vi "Live.vi"(1 "baud rate (9600)":u32=9600, 2 "VISA Resource (read)":refnum<visa-resource-name>="COM2") -> (0 "CAR DATA":T1)   [LabVIEW 2014]
uses:
  Program Files (x86)/National Instruments/LabVIEW 2014/examples/Instrument IO/Serial/support/Serial - Settings.ctl
  Type Def/CAR Data Cluster.ctl
  <vilib>/Instr/_visa.llb/VISA Configure Serial Port (Instr).vi
panel:
  in  "Termination Character":u8=10 format="%.0x"
  in  "End Write on Termination Character?":bool=TRUE
  in  "End Read on Termination Character?":bool=TRUE
  in  "Write String":string="*IDN?"
  in  "Serial Settings (read)":T2={"baud rate"=9600, "data bits"=8, "parity"=enum."None", "stop bits"=10, "flow control"=0} {"flow control" items=["None"=0, "XON/XOFF"=1, "RTS/CTS"=2, "DTR/DSR"=4]; "stop bits" items=["1.0"=10, "1.5"=15, "2.0"=20]; "data bits" min=5 max=8 step=1; "baud rate" items=["75"=75, "110"=110, "134"=134, "150"=150, "300"=300, "600"=600, "1200"=1200, "1800"=1800, "2400"=2400, "4800"=4800, "7200"=7200, "9600"=9600, "14400"=14400, "19200"=19200, "28800"=28800, "38400"=38400, "56000"=56000, "57600"=57600, "115200"=115200, "128000"=128000, "230400"=230400]}
  in  "Serial Settings (write)":T2={"baud rate"=9600, "data bits"=8, "parity"=enum."None", "stop bits"=10, "flow control"=0} {"flow control" items=["None"=0, "XON/XOFF"=1, "RTS/CTS"=2, "DTR/DSR"=4]; "stop bits" items=["1.0"=10, "1.5"=15, "2.0"=20]; "data bits" min=5 max=8 step=1; "baud rate" items=["75"=75, "110"=110, "134"=134, "150"=150, "300"=300, "600"=600, "1200"=1200, "1800"=1800, "2400"=2400, "4800"=4800, "7200"=7200, "9600"=9600, "14400"=14400, "19200"=19200, "28800"=28800, "38400"=38400, "56000"=56000, "57600"=57600, "115200"=115200, "128000"=128000, "230400"=230400]}
  in  "VISA Resource (write)":refnum<visa-resource-name>="COM1"
  out "bytes written":u32
  out "Read String":string
  out "bytes read":u32
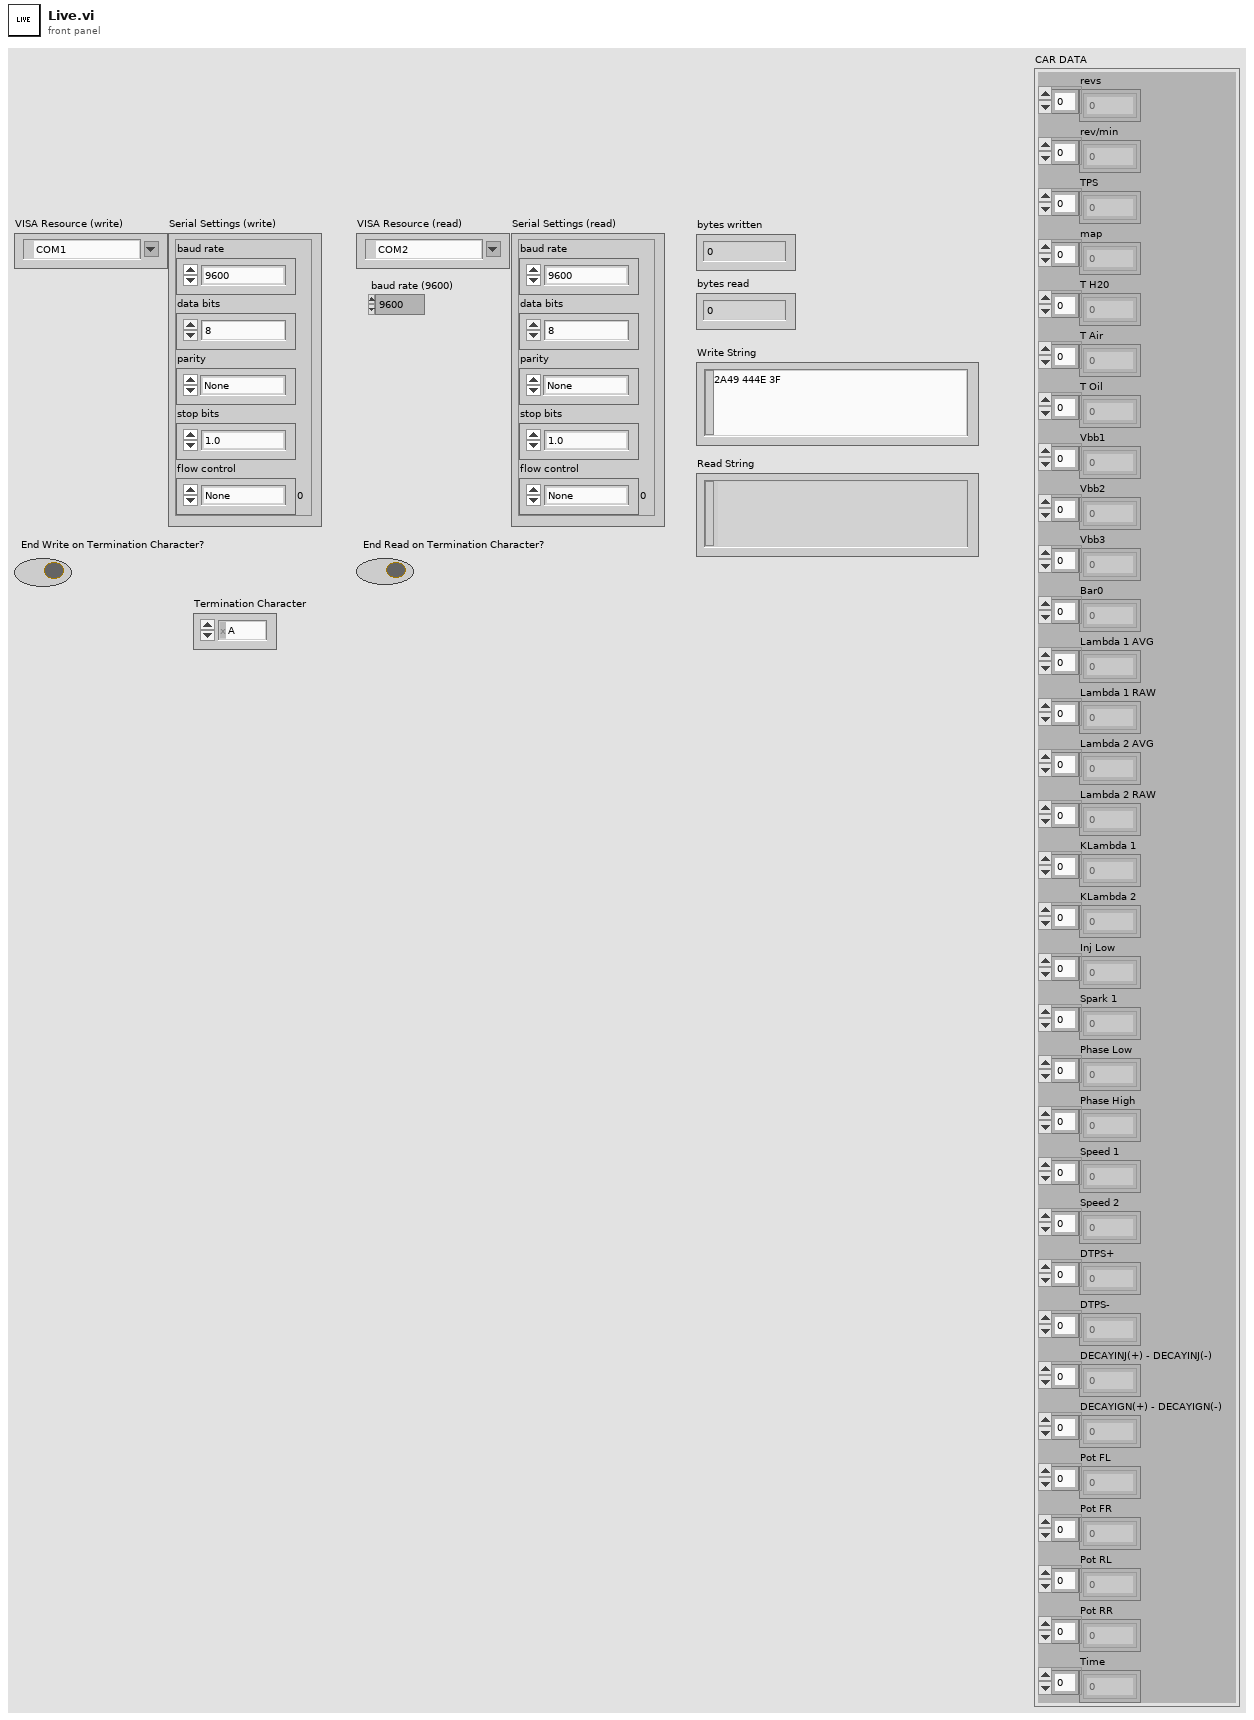
[diagram p1: front panel]
types:
  T1 = typedef "CAR Data Cluster.ctl" = cluster{"revs":dbl[], "rev/min":dbl[], "TPS":dbl[], "map":dbl[], "T H20":dbl[], "T Air":dbl[], "T Oil":dbl[], "Vbb1":dbl[], "Vbb2":dbl[], "Vbb3":dbl[], "Bar0":dbl[], "Lambda 1 AVG":dbl[], "Lambda 1 RAW":dbl[], "Lambda 2 AVG":dbl[], "Lambda 2 RAW":dbl[], "KLambda 1":dbl[], "KLambda 2":dbl[], "Inj Low":dbl[], "Spark 1":dbl[], "Phase Low":dbl[], "Phase High":dbl[], "Speed 1":dbl[], "Speed 2":dbl[], "DTPS+":dbl[], "DTPS-":dbl[], "DECAYINJ(+) - DECAYINJ(-)":dbl[], "DECAYIGN(+) - DECAYIGN(-)":dbl[], "Pot FL":dbl[], "Pot FR":dbl[], "Pot RL":dbl[], "Pot RR":dbl[], "Time":dbl[]}
  T2 = typedef "Serial - Settings.ctl" = cluster{"baud rate":u32, "data bits":u16, "parity":enum16{"None", "Odd", "Even", "Mark", "Space"}, "stop bits":u16, "flow control":u16}
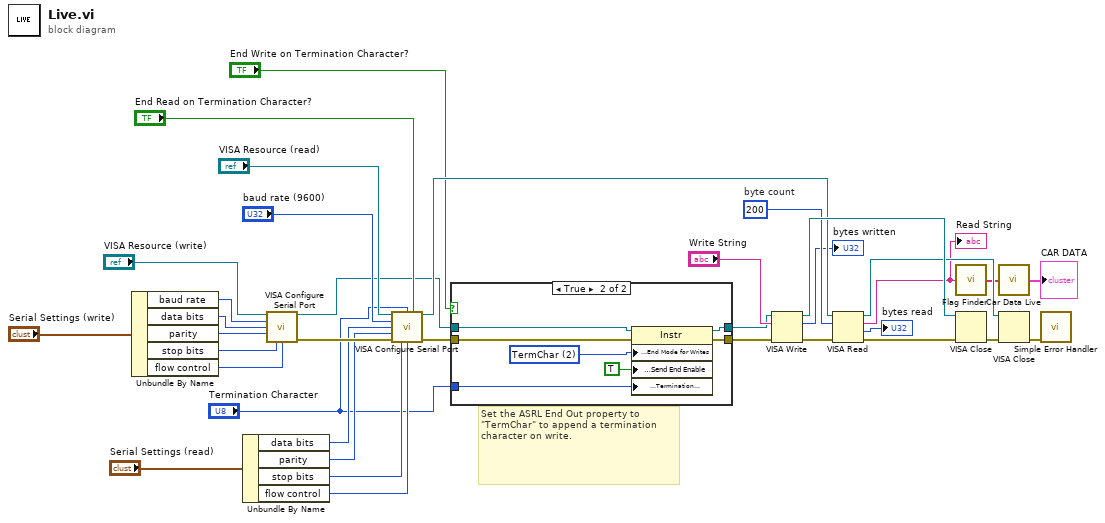
[diagram p0: block diagram]
diagram:
  w31 = u32 200  # byte count
  # "Set the ASRL End Out property to \"TermChar\" to append a termination character on write."
  n1 = Unbundle By Name("Serial Settings (write)") -> ("baud rate"=w22:u32, "data bits"=w21:u16, "parity"=w20:enum16{"None", "Odd", "Even", "Mark", "Space"}, "stop bits"=w19:u16, "flow control"=w18:u16)
  n2 = Unbundle By Name("Serial Settings (read)") -> ("data bits"=w15:u16, "parity"=w14:enum16{"None", "Odd", "Even", "Mark", "Space"}, "stop bits"=w13:u16, "flow control"=w12:u16)
  n3 = call-poly "VISA Configure Serial Port"("VISA resource name"="VISA Resource (write)", "baud rate (9600)"=w22, "data bits (8)"=w21, "parity (0:none)"=w20, "stop bits (10: 1 bit)"=w19, "flow control (0:none)"=w18) -> ("VISA resource name out"=w9:refnum<visa-resource-name>, "error out"=w28:errorcluster)  [unwired: 3 in, 5 out]
  n4 = call-poly "VISA Configure Serial Port"("VISA resource name"="VISA Resource (read)", "termination char\n(0xA = '\\n' = LF)"="Termination Character", "Enable Termination\nChar (T)"="End Read on Termination Character?", "baud rate (9600)"="baud rate (9600)", "data bits (8)"=w15, "parity (0:none)"=w14, "error in (no error)"=w28, "stop bits (10: 1 bit)"=w13, "flow control (0:none)"=w12) -> ("VISA resource name out"=w34:refnum<visa-resource-name>, "error out"=w7:errorcluster)  [unwired: 1 in, 4 out]
  n5 = case shown="True" "End Write on Termination Character?" {
    tunnel: w9 -> [w37 w45]
    tunnel: w7 -> [w38 w44]
    tunnel: [w37 w43] -> w8
    tunnel: [w38 w42] -> w6
    tunnel: "Termination Character" -> [_ w40]
    frame False {
    }
    frame True {
      w41 = u16 2 items=["None", "LastBit", "TermChar", "Break"] ("Serial Settings:Serial End Mode for Writes")
      n6 = property class="Instr"(reference=w45, error in=w44, "Serial Settings:End Mode for Writes"=w41, "Message Based Settings:Send End Enable"=TRUE, "Message Based Settings:Termination Character"=w40) -> (reference out=w43:refnum<visa-resource-name>, error out=w42:errorcluster)
    }
  }
  n7 = VISA Write(VISA resource name=w8, write buffer="Write String", error in (no error)=w6) -> (VISA resource name out=w35:refnum<visa-resource-name>, return count=→"bytes written":u32, error out=w27:errorcluster)
  n8 = VISA Read(VISA resource name=w34, byte count=w31, error in (no error)=w27) -> (VISA resource name out=w33:refnum<visa-resource-name>, read buffer=w3:string, return count=→"bytes read":u32, error out=w26:errorcluster)
  "Read String" <- w3
  n9 = call "Flag Finder.vi"("read buffer"=w3) -> ("Output Array"=w2:string[])  [unwired: 4 in]
  n10 = VISA Close(VISA resource name=w35, error in (no error)=w26) -> (error out=w25:errorcluster)
  n11 = call "Car Data Live.vi"("Input Array"=w2) -> ("CAR DATA"=→"CAR DATA":T1)
  n12 = VISA Close(VISA resource name=w33, error in (no error)=w25) -> (error out=w24:errorcluster)
  n13 = call <vilib>:"Simple Error Handler.vi"("error in (no error)"=w24) -> ()  [unwired: 1 in, 8 out]
